vi "Find Red Pitaya Digitizers VISA.vi"(6 "Timeout":i32=100, 7 "Logic tags":u16[](array[numeric])=[101, 102], 8 "Error In":errorcluster, 9 "End address":i32=120, 10 "Start address":i32=100, 11 "Subnet":string="192.168.1") -> (0 "Error Out":errorcluster, 1 "connections":refnum<visa-resource-name>[](array[refnum]), 2 "Device names":string[](array[string]), 3 "Digitizers out":refnum<class "Pulse Driver.lvclass">[](array[class]))   [LabVIEW 2024]
uses:
  Red Pitaya Digitizer.lvclass
  RP Core/RP Instrument/RP Instrument.lvclass
  D:/GitHub/NHMFL_Core/Libraries/Instruments/Pulse Driver/Lockin Digitizer Driver/Lockin Digitizer Driver.lvclass
  D:/GitHub/NHMFL_Core/Libraries/Instruments/Pulse Driver/Pulse Driver.lvclass
  D:/GitHub/NHMFL_Core/Libraries/Instruments/Simple VISA Reader/Simple VISA Reader Driver.lvclass
  D:/GitHub/NHMFL_Core/Libraries/Instruments/VISA Instrument/VISA Instrument.lvclass
  D:/GitHub/NHMFL_Core/Libraries/Instruments/Instrument Driver/Instrument Driver.lvclass
  D:/GitHub/NHMFL_Core/Libraries/Red Pitaya/Red Pitaya Digitizer/Red Pitaya Digitizer.lvclass
  Instruments/Pulse Driver/Pulse Driver.lvclass
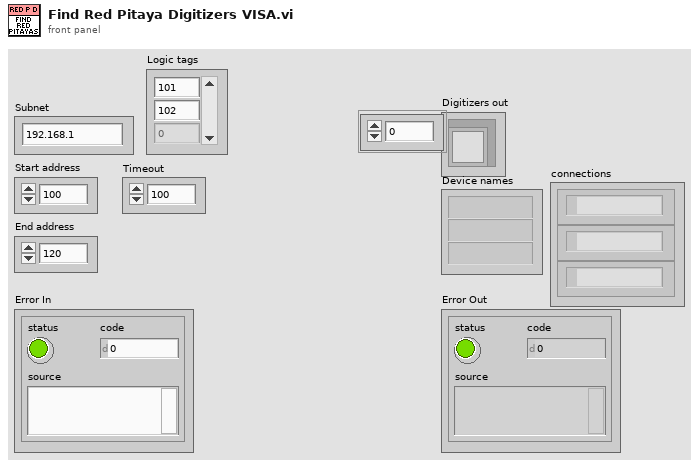
[diagram p1: front panel]
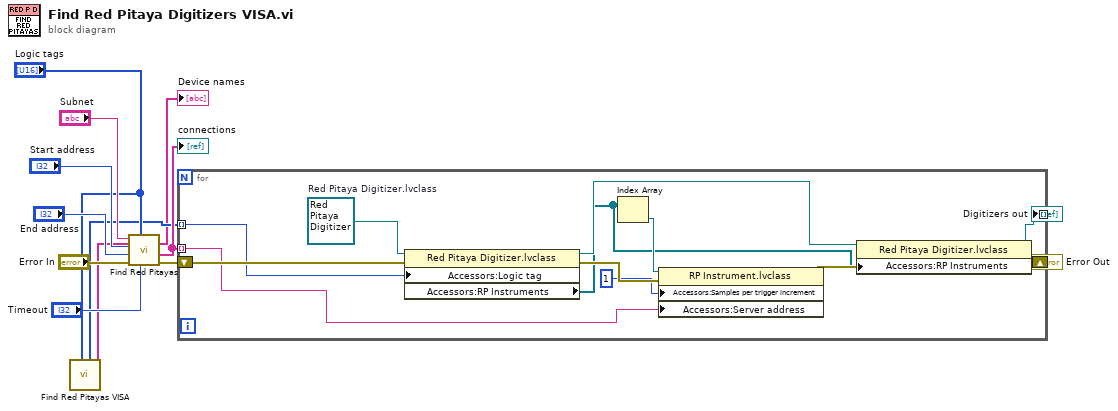
[diagram p0: block diagram]
diagram:
  n1 = call "Find Red Pitayas VISA.vi"("Logic tags"="Logic tags") -> ("Device names"=→"Device names":string[], "Logic tags out"=w2:u16[])  [unwired: 7 in, 2 out]
  n2 = call "Find Red Pitayas.vi"("Timeout"="Timeout", "Acceptable logic tags"="Logic tags", "Error In"="Error In", "End address"="End address", "Start address"="Start address", "Subnet"="Subnet") -> ("Error Out"=w4:errorcluster, "Addresses"=w6:string[])  [unwired: 4 out]
  "connections" <- w6
  n3 = for {
    tunnel: w6 -> [w15] mode=indexing
    shift-right: [w20] -> w12
    shift-left: w4 -> [w23]
    tunnel: [w17] -> w11 mode=indexing
    tunnel: w2 -> [w16] mode=indexing
    w24 = refnum<class "Red Pitaya Digitizer.lvclass"> refnum  # Red Pitaya Digitizer.lvclass
    n4 = property class="Red Pitaya Digitizer.lvclass"(reference=w24, error in=w23, "Accessors:Logic tag"=w16) -> (reference out=w18:refnum<class "Red Pitaya Digitizer.lvclass">, error out=w22:errorcluster, "Accessors:RP Instruments"=w13:refnum<class "RP Instrument.lvclass">[])
    n5 = Index Array(array=w13) -> (element=w14:refnum<class "RP Instrument.lvclass">)  [unwired: 1 in]
    n6 = property class="RP Instrument.lvclass"(reference=w14, error in=w22, "Accessors:Samples per trigger increment "=1 ("Samples per trigger increment"), "Accessors:Server address"=w15) -> (error out=w19:errorcluster)  [unwired: 1 out]
    n7 = property class="Red Pitaya Digitizer.lvclass"(reference=w18, error in=w19, "Accessors:RP Instruments"=w13) -> (reference out=w17:refnum<class "Red Pitaya Digitizer.lvclass">, error out=w20:errorcluster)
  }
  "Digitizers out" <- w11
  "Error Out" <- w12
